vi "表格翻页.vi"() -> ()   [LabVIEW 2014]
doc: "该VI是LabVIEW核心课程1中练习的答案。\n\n该VI使用While循环和移位寄存器进行均值计算。无需硬件。"
panel:
  in  "下一页":bool
  in  "上一页":bool
  out "表格控件":string[][](table)
  in  "停止按钮":bool
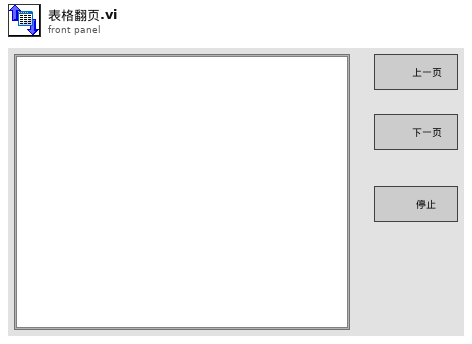
[diagram p1: front panel]
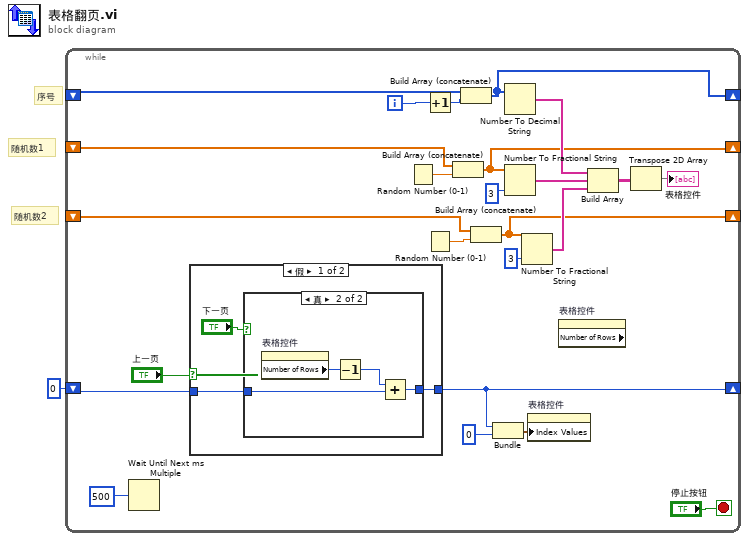
[diagram p0: block diagram]
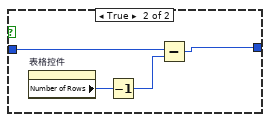
[diagram p3: hidden frame]
diagram:
  # "随机数2"
  # "随机数1"
  # "序号"
  n1 = while {
    shift-right: [w16] -> _
    shift-left: _ -> [w15]
    shift-right: [w14] -> _
    shift-left: _ -> [w13]
    shift-right: [w12] -> _
    shift-left: _ -> [w11]
    shift-right: [w7] -> _
    shift-left: 0 -> [w6]
    i -> [w4]
    stop <- "停止按钮" stop-if-true
    n2 = Wait Until Next ms Multiple ("等待下一个整数倍毫秒")(millisecond multiple=u32 500) -> ()  [unwired: 1 out]
    n3 = case shown="假" "上一页" {
      tunnel: [w28 w36] -> w7
      tunnel: w6 -> [w26 w37]
      frame False {
        n4 = case shown="真" "下一页" {
          tunnel: w26 -> [w29 w33]
          tunnel: [w29 w32] -> w28
          frame False {
          }
          frame True {
            n5 = property on="表格控件" class="Tbl (严格)"() -> ("Number of Rows"=w31:u32)  [unwired: 2 in, 2 out]
            n6 = Decrement(x=w31) -> (x-1=w30:u32)
            n7 = Add(x=w30, y=w33) -> (x+y=w32:u32)
          }
        }
      }
      frame True {
        n8 = property on="表格控件" class="Tbl (严格)"() -> ("Number of Rows"=w35:u32)  [unwired: 2 in, 2 out]
        n9 = Decrement(x=w35) -> (x-1=w34:u32)
        n10 = Subtract(x=w37, y=w34) -> (x-y=w36:u32)
      }
    }
    n11 = Random Number (0-1)() -> (number: 0 to 1=w3:dbl)
    n12 = Increment(x=w4) -> (x+1=w17:i32)
    n13 = Random Number (0-1)() -> (number: 0 to 1=w2:dbl)
    n14 = Build Array (concatenate)(w15, w3) -> (w16:dbl[])
    n15 = Build Array (concatenate)(w11, w17) -> (w12:i32[])
    n16 = Build Array (concatenate)(w13, w2) -> (w14:dbl[])
    n17 = Bundle(w7, 0) -> (w9:cluster{u32, i32})  [unwired: 1 in]
    n18 = Number To Decimal String(number=w12) -> (decimal integer string=w21:string[])  [unwired: 1 in]
    n19 = Number To Fractional String(number=w16, precision (6)=i16 3 ("精度(6)")) -> (F-format string=w20:string[])  [unwired: 2 in]
    n20 = Number To Fractional String(number=w14, precision (6)=i16 3 ("精度(6)")) -> (F-format string=w22:string[])  [unwired: 2 in]
    n21 = property on="表格控件" class="Tbl (严格)"("Index Values"=w9) -> ()  [unwired: 2 in, 2 out]
    n22 = property on="表格控件" class="Tbl (严格)" props=["Number of Rows"]() -> ()  [unwired: 2 in, 3 out]
    n23 = Build Array(w21, w20, w22) -> (w19:string[][])
    n24 = Transpose 2D Array(2D array=w19) -> (transposed array=→"表格控件":string[][])
  }
